vi "CRYInsert All to Listbox.vi"(11 "sAction":string) -> ()   [LabVIEW 2013]
uses:
  Global/CRYCurve Library Global.vi
panel:
  # "Insert All(Curve, Value, Result, Waveform) to Listbox"
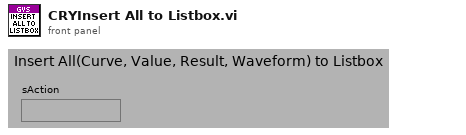
[diagram p1: front panel]
types:
  T1 = cluster{"Left Cell String":string, "Child Text":string[], "Child Tag":string, "Item Indent":i32, "Child Only?":bool, "Glyph Index":i32}[]
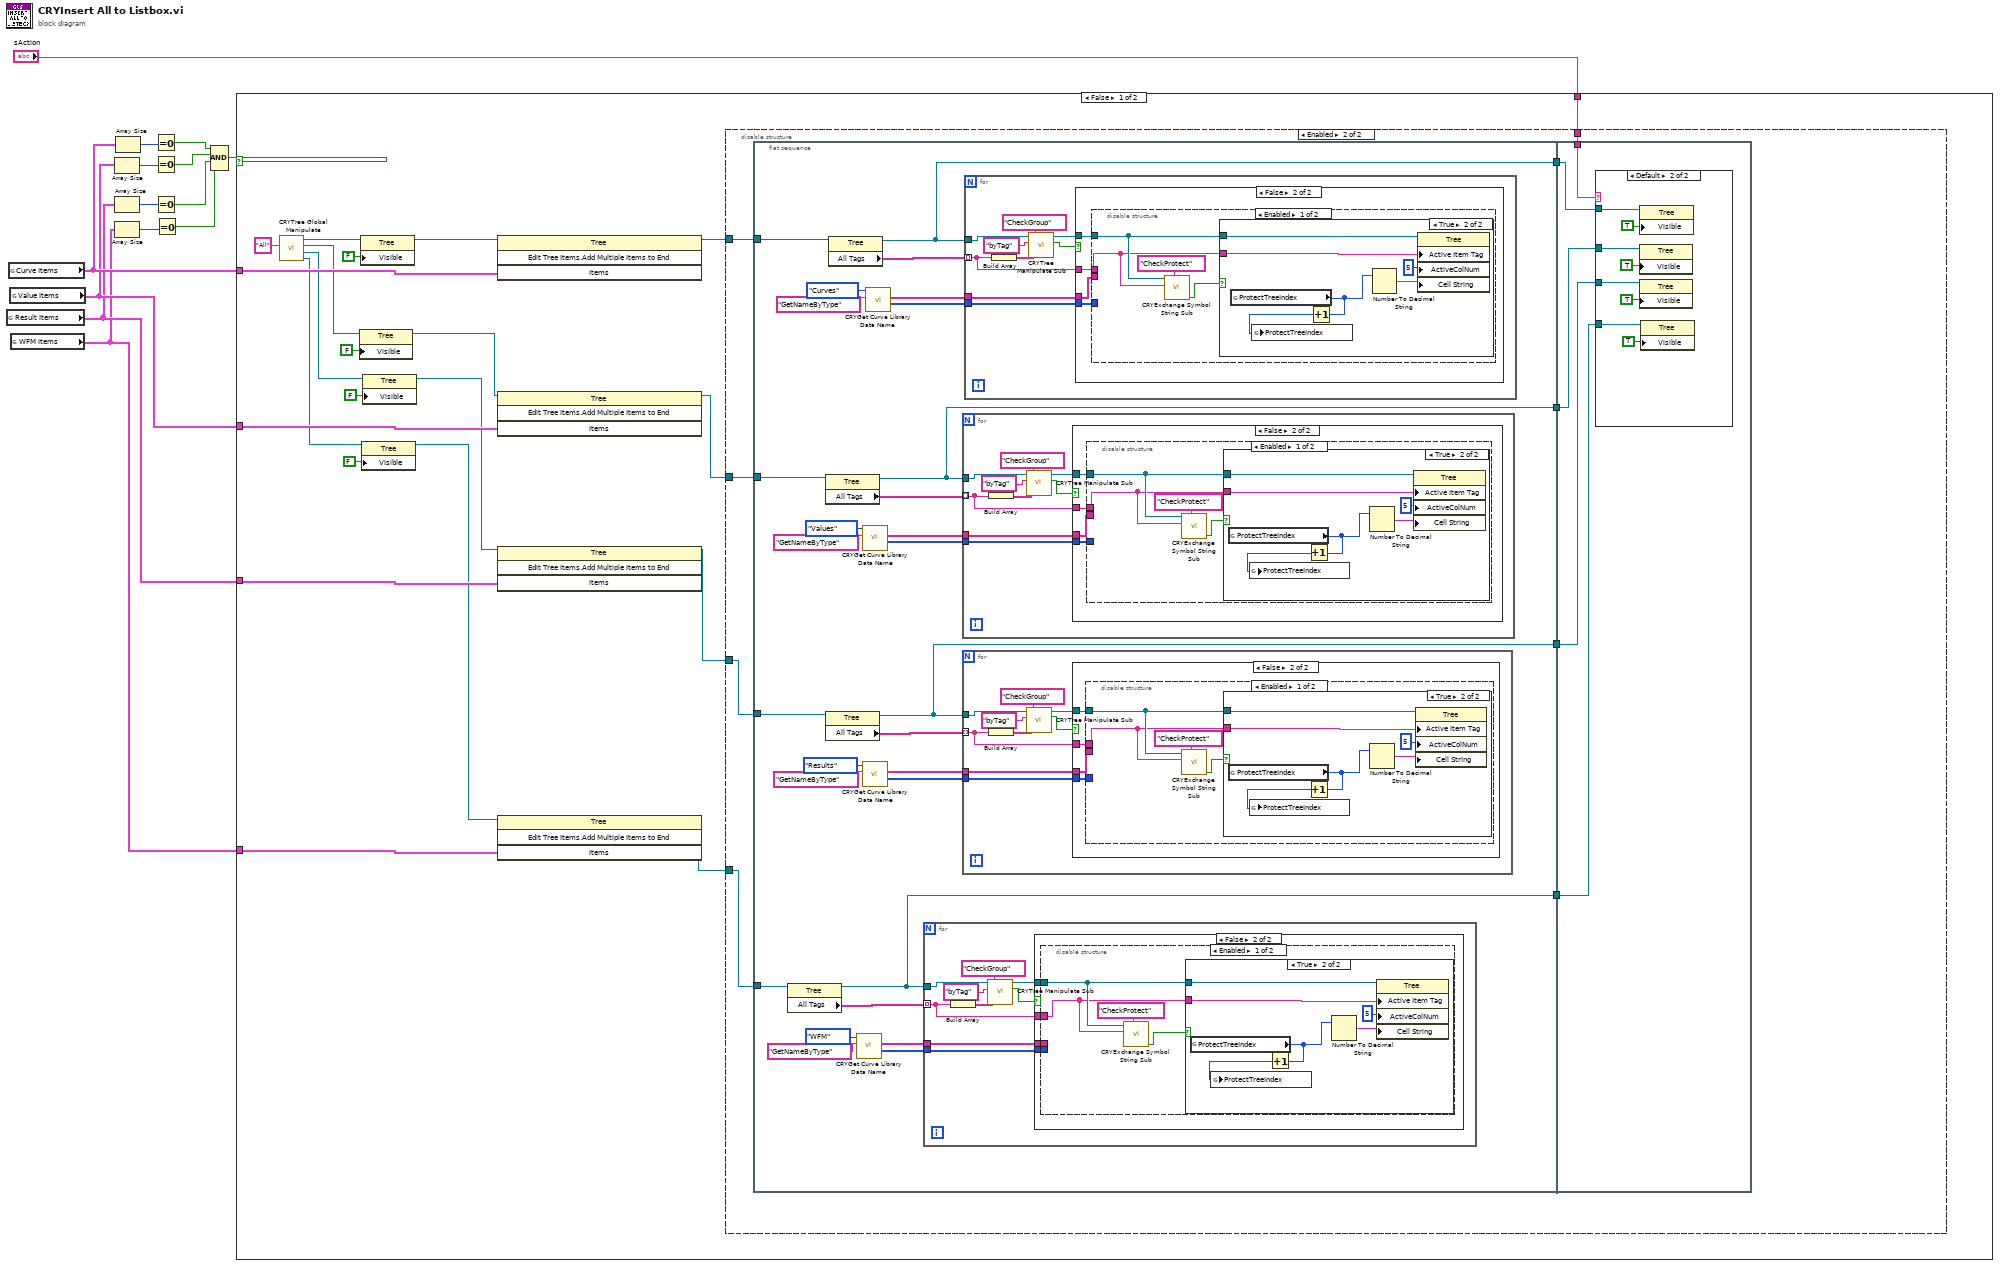
[diagram p0: block diagram]
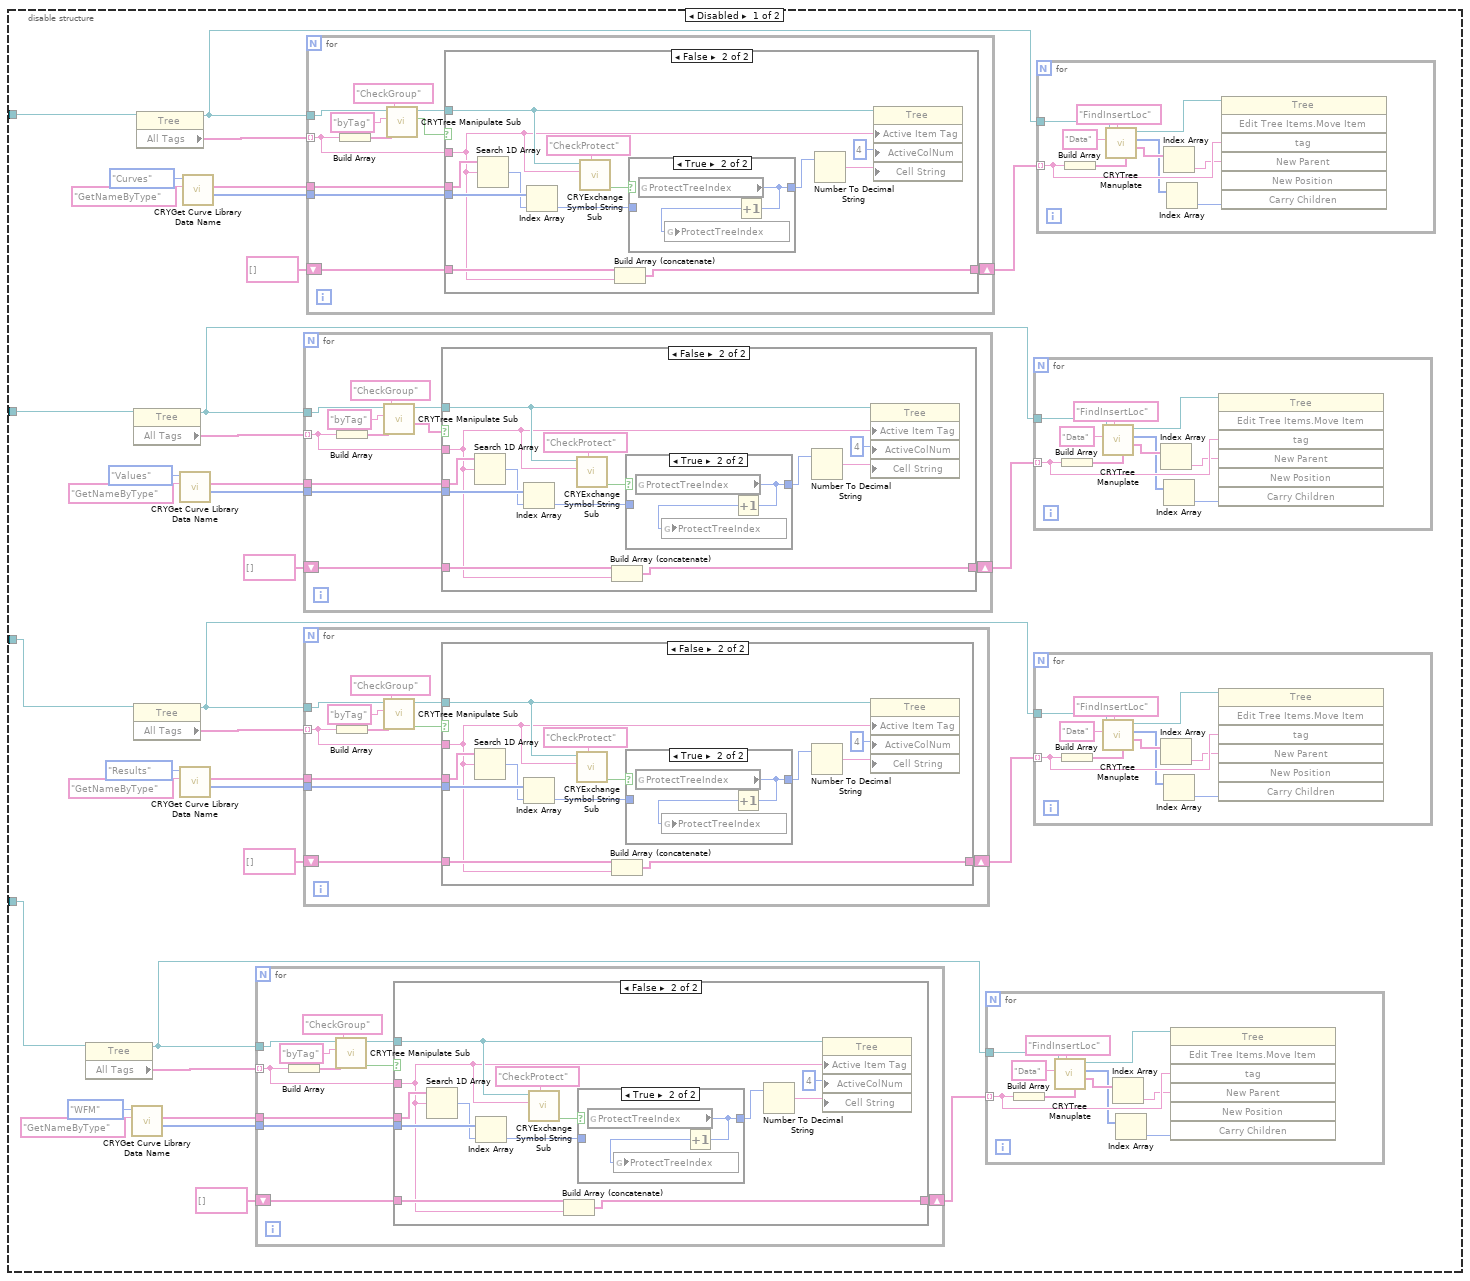
[diagram p2: hidden frame]
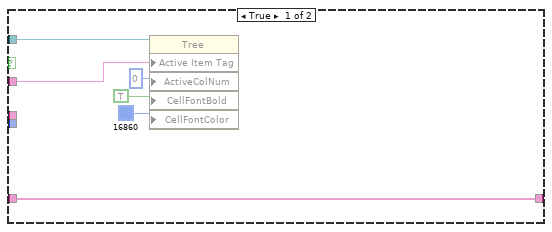
[diagram p3: hidden frame]
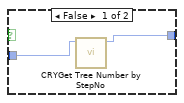
[diagram p4: hidden frame]
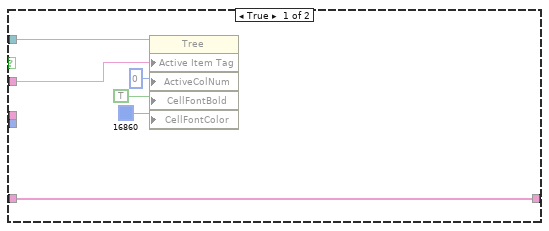
[diagram p5: hidden frame]
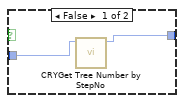
[diagram p6: hidden frame]
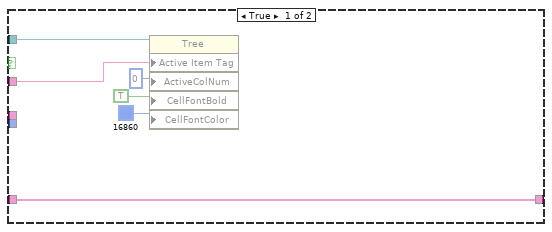
[diagram p7: hidden frame]
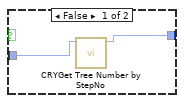
[diagram p8: hidden frame]
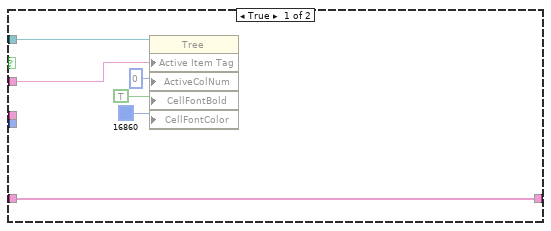
[diagram p9: hidden frame]
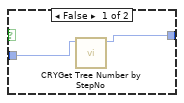
[diagram p10: hidden frame]
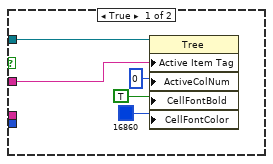
[diagram p11: hidden frame]
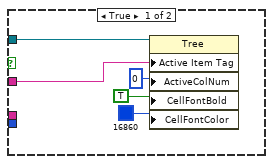
[diagram p14: hidden frame]
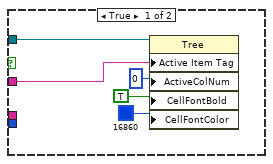
[diagram p17: hidden frame]
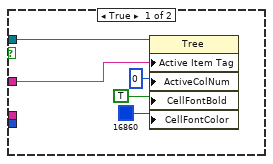
[diagram p20: hidden frame]
diagram:
  n1 = global read "CRYCurve Library Global.vi" "Result Items"() -> (w12:T1)
  n2 = global read "CRYCurve Library Global.vi" "Curve Items"() -> (w14:T1)
  n3 = global read "CRYCurve Library Global.vi" "Value Items"() -> (w13:T1)
  n4 = global read "CRYCurve Library Global.vi" "WFM Items"() -> (w11:T1)
  n5 = Array Size(array=w13) -> (size(s)=w9:i32)
  n6 = Array Size(array=w12) -> (size(s)=w8:i32)
  n7 = Array Size(array=w11) -> (size(s)=w7:i32)
  n8 = Array Size(array=w14) -> (size(s)=w10:i32)
  n9 = Equal To 0?(x=w10) -> (x = 0?=w6:bool)
  n10 = Equal To 0?(x=w9) -> (x = 0?=w4:bool)
  n11 = Equal To 0?(x=w8) -> (x = 0?=w5:bool)
  n12 = Equal To 0?(x=w7) -> (x = 0?=w3:bool)
  n13 = Compound Arithmetic op=AND(w6, w4, w5, w3) -> (w2:bool)
  n14 = case shown="False" w2 {
    tunnel: w14 -> [w31 _]
    tunnel: w13 -> [w30 _]
    tunnel: w12 -> [w29 _]
    tunnel: w11 -> [w28 _]
    tunnel: "sAction" -> [w15 _]
    frame False {
      n15 = call "CRYTree Global Manipulate.vi"("sOption"="All") -> ("WFM Tree"=w18:refnum<vi>, "Results Tree"=w20:refnum<vi>, "Values Tree"=w23:refnum<vi>, "Tree/Curve Tree"=w27:refnum<vi>)  [unwired: 7 in]
      n16 = property class="Tree"(reference=w23, "Visible"=FALSE) -> (reference out=w22:refnum<vi>)  [unwired: 1 in, 1 out]
      n17 = property class="Tree"(reference=w27, "Visible"=FALSE) -> (reference out=w26:refnum<vi>)  [unwired: 1 in, 1 out]
      n18 = property class="Tree"(reference=w18, "Visible"=FALSE) -> (reference out=w16:refnum<vi>)  [unwired: 1 in, 1 out]
      n19 = property class="Tree"(reference=w20, "Visible"=FALSE) -> (reference out=w17:refnum<vi>)  [unwired: 1 in, 1 out]
      n20 = invoke class="Tree" method="Edit Tree Items.Add Multiple Items to End"(reference=w26, "Items"=w31) -> (reference out=w36:refnum<vi>)  [unwired: 2 in, 3 out]
      n21 = invoke class="Tree" method="Edit Tree Items.Add Multiple Items to End"(reference=w22, "Items"=w30) -> (reference out=w33:refnum<vi>)  [unwired: 2 in, 3 out]
      n22 = invoke class="Tree" method="Edit Tree Items.Add Multiple Items to End"(reference=w17, "Items"=w29) -> (reference out=w34:refnum<vi>)  [unwired: 2 in, 3 out]
      n23 = invoke class="Tree" method="Edit Tree Items.Add Multiple Items to End"(reference=w16, "Items"=w28) -> (reference out=w35:refnum<vi>)  [unwired: 2 in, 3 out]
      n24 = disable-structure shown="Enabled" {
        disable-tunnel: w36 -> [w70 w257]
        disable-tunnel: w35 -> [w37 w254]
        disable-tunnel: w34 -> [w46 w255]
        disable-tunnel: w33 -> [w55 w256]
        disable-tunnel: w15 -> [_ w252]
        frame Disabled {
          n25 = property class="Tree"(reference=w37) -> (reference out=w39:refnum<vi>, "All Tags"=w40:string[])  [unwired: 1 in, 1 out]
          n26 = call "CRYGet Curve Library Data Name.vi"("sAction"="GetNameByType", "Type"=enum16{"Curves", "Values", "Results", "WFM"}."WFM") -> ("nStep No"=w43:i32[], "sNames"=w42:string[])  [unwired: 6 in, 2 out]
          n27 = property class="Tree"(reference=w55) -> (reference out=w57:refnum<vi>, "All Tags"=w58:string[])  [unwired: 1 in, 1 out]
          n28 = property class="Tree"(reference=w46) -> (reference out=w48:refnum<vi>, "All Tags"=w49:string[])  [unwired: 1 in, 1 out]
          n29 = property class="Tree"(reference=w70) -> (reference out=w71:refnum<vi>, "All Tags"=w69:string[])  [unwired: 1 in, 1 out]
          n30 = call "CRYGet Curve Library Data Name.vi"("sAction"="GetNameByType", "Type"=enum16{"Curves", "Values", "Results", "WFM"}."Values") -> ("nStep No"=w61:i32[], "sNames"=w60:string[])  [unwired: 6 in, 2 out]
          n31 = call "CRYGet Curve Library Data Name.vi"("sAction"="GetNameByType", "Type"=enum16{"Curves", "Values", "Results", "WFM"}."Results") -> ("nStep No"=w52:i32[], "sNames"=w51:string[])  [unwired: 6 in, 2 out]
          n32 = call "CRYGet Curve Library Data Name.vi"("sAction"="GetNameByType", "Type"=enum16{"Curves", "Values", "Results", "WFM"}."Curves") -> ("nStep No"=w66:i32[], "sNames"=w67:string[])  [unwired: 6 in, 2 out]
          n33 = for {
            tunnel: w40 -> [w87] mode=indexing
            tunnel: w39 -> [w91]
            tunnel: w42 -> [w86]
            tunnel: w43 -> [w85]
            shift-right: [w83] -> w38
            shift-left: string[] [] ("sNames") -> [w84]
            n34 = Build Array(w87) -> (w90:string[])
            n35 = call "CRYTree Manipulate Sub.vi"("sAction"="CheckGroup", "sData"=w90, "sOption"="byTag", "Tree in"=w91) -> ("bData out"=w89:bool, "Tree Out"=w88:refnum<vi>)  [unwired: 3 in, 3 out]
            n36 = case shown="False" w89 {
              tunnel: w88 -> [w96 w101]
              tunnel: w87 -> [w95 w100]
              tunnel: w86 -> [_ w110]
              tunnel: w85 -> [_ w109]
              tunnel: w84 -> [w94 w107]
              tunnel: [w94 w106] -> w83
              frame True {
                n37 = property class="Tree"(reference=w96, "Active Item Tag"=w95, "ActiveColNum"=0 ("Active Cell:Active Column Number"), "CellFontBold"=TRUE ("Active Cell:Cell Font:Bold"), "CellFontColor"=u32 16860) -> ()  [unwired: 1 in, 2 out]
              }
              frame False {
                n38 = Search 1D Array(1D array=w110, element=w100) -> (index of element=w108:i32)  [unwired: 1 in]
                n39 = Index Array(array=w109, index=w108) -> (element=w102:i32)
                n40 = call "CRYExchange Symbol String Sub.vi"("sAction"="CheckProtect", "sData"=w100, "Tree in"=w101) -> ("bData Out"=w105:bool)  [unwired: 5 in, 3 out]
                n41 = Build Array (concatenate)(w107, w100) -> (w106:string[])
                n42 = case shown="True" w105 {
                  tunnel: [w114 w115] -> w103
                  tunnel: w102 -> [w113 _]
                  frame False {
                    n43 = call "CRYGet Tree Number by StepNo.vi"("Step Setup VI No"=w113) -> ("Number in Tree"=w114:i32)  [unwired: 9 in, 1 out]
                  }
                  frame True {
                    n44 = global read "CRYCurve Library Global.vi" "ProtectTreeIndex"() -> (w115:i32)
                    n45 = Increment(x=w115) -> (x+1=w116:i32)
                    n46 = global write "CRYCurve Library Global.vi" "ProtectTreeIndex"(w116) -> ()
                  }
                }
                n47 = Number To Decimal String(number=w103) -> (decimal integer string=w111:string)  [unwired: 1 in]
                n48 = property class="Tree"(reference=w101, "Active Item Tag"=w100, "ActiveColNum"=4 ("Active Cell:Active Column Number"), "Cell String"=w111) -> ()  [unwired: 1 in, 2 out]
              }
            }
          }
          n49 = for {
            tunnel: w58 -> [w176] mode=indexing
            tunnel: w57 -> [w179]
            tunnel: w60 -> [w175]
            tunnel: w61 -> [w174]
            shift-right: [w172] -> w56
            shift-left: string[] [] ("sNames") -> [w173]
            n50 = Build Array(w176) -> (w178:string[])
            n51 = call "CRYTree Manipulate Sub.vi"("sAction"="CheckGroup", "sData"=w178, "sOption"="byTag", "Tree in"=w179) -> ("sData Out"=w171:string[], "Tree Out"=w177:refnum<vi>)  [unwired: 3 in, 3 out]
            n52 = case shown="False" w171 {
              tunnel: w177 -> [w184 w189]
              tunnel: w176 -> [w183 w188]
              tunnel: w175 -> [_ w198]
              tunnel: w174 -> [_ w197]
              tunnel: w173 -> [w182 w195]
              tunnel: [w182 w194] -> w172
              frame True {
                n53 = property class="Tree"(reference=w184, "Active Item Tag"=w183, "ActiveColNum"=0 ("Active Cell:Active Column Number"), "CellFontBold"=TRUE ("Active Cell:Cell Font:Bold"), "CellFontColor"=u32 16860) -> ()  [unwired: 1 in, 2 out]
              }
              frame False {
                n54 = Search 1D Array(1D array=w198, element=w188) -> (index of element=w196:i32)  [unwired: 1 in]
                n55 = Index Array(array=w197, index=w196) -> (element=w190:i32)
                n56 = call "CRYExchange Symbol String Sub.vi"("sAction"="CheckProtect", "sData"=w188, "Tree in"=w189) -> ("bData Out"=w193:bool)  [unwired: 5 in, 3 out]
                n57 = Build Array (concatenate)(w195, w188) -> (w194:string[])
                n58 = case shown="True" w193 {
                  tunnel: [w202 w203] -> w191
                  tunnel: w190 -> [w201 _]
                  frame False {
                    n59 = call "CRYGet Tree Number by StepNo.vi"("Step Setup VI No"=w201) -> ("Number in Tree"=w202:i32)  [unwired: 9 in, 1 out]
                  }
                  frame True {
                    n60 = global read "CRYCurve Library Global.vi" "ProtectTreeIndex"() -> (w203:i32)
                    n61 = Increment(x=w203) -> (x+1=w204:i32)
                    n62 = global write "CRYCurve Library Global.vi" "ProtectTreeIndex"(w204) -> ()
                  }
                }
                n63 = Number To Decimal String(number=w191) -> (decimal integer string=w199:string)  [unwired: 1 in]
                n64 = property class="Tree"(reference=w189, "Active Item Tag"=w188, "ActiveColNum"=4 ("Active Cell:Active Column Number"), "Cell String"=w199) -> ()  [unwired: 1 in, 2 out]
              }
            }
          }
          n65 = for {
            tunnel: w49 -> [w131] mode=indexing
            tunnel: w48 -> [w135]
            tunnel: w51 -> [w130]
            tunnel: w52 -> [w129]
            shift-right: [w127] -> w47
            shift-left: string[] [] ("sNames") -> [w128]
            n66 = Build Array(w131) -> (w134:string[])
            n67 = call "CRYTree Manipulate Sub.vi"("sAction"="CheckGroup", "sData"=w134, "sOption"="byTag", "Tree in"=w135) -> ("bData out"=w133:bool, "Tree Out"=w132:refnum<vi>)  [unwired: 3 in, 3 out]
            n68 = case shown="False" w133 {
              tunnel: w132 -> [w140 w145]
              tunnel: w131 -> [w139 w144]
              tunnel: w130 -> [_ w154]
              tunnel: w129 -> [_ w153]
              tunnel: w128 -> [w138 w151]
              tunnel: [w138 w150] -> w127
              frame True {
                n69 = property class="Tree"(reference=w140, "Active Item Tag"=w139, "ActiveColNum"=0 ("Active Cell:Active Column Number"), "CellFontBold"=TRUE ("Active Cell:Cell Font:Bold"), "CellFontColor"=u32 16860) -> ()  [unwired: 1 in, 2 out]
              }
              frame False {
                n70 = Search 1D Array(1D array=w154, element=w144) -> (index of element=w152:i32)  [unwired: 1 in]
                n71 = Index Array(array=w153, index=w152) -> (element=w146:i32)
                n72 = call "CRYExchange Symbol String Sub.vi"("sAction"="CheckProtect", "sData"=w144, "Tree in"=w145) -> ("bData Out"=w149:bool)  [unwired: 5 in, 3 out]
                n73 = Build Array (concatenate)(w151, w144) -> (w150:string[])
                n74 = case shown="True" w149 {
                  tunnel: [w158 w159] -> w147
                  tunnel: w146 -> [w157 _]
                  frame False {
                    n75 = call "CRYGet Tree Number by StepNo.vi"("Step Setup VI No"=w157) -> ("Number in Tree"=w158:i32)  [unwired: 9 in, 1 out]
                  }
                  frame True {
                    n76 = global read "CRYCurve Library Global.vi" "ProtectTreeIndex"() -> (w159:i32)
                    n77 = Increment(x=w159) -> (x+1=w160:i32)
                    n78 = global write "CRYCurve Library Global.vi" "ProtectTreeIndex"(w160) -> ()
                  }
                }
                n79 = Number To Decimal String(number=w147) -> (decimal integer string=w155:string)  [unwired: 1 in]
                n80 = property class="Tree"(reference=w145, "Active Item Tag"=w144, "ActiveColNum"=4 ("Active Cell:Active Column Number"), "Cell String"=w155) -> ()  [unwired: 1 in, 2 out]
              }
            }
          }
          n81 = for {
            tunnel: w69 -> [w220] mode=indexing
            tunnel: w71 -> [w223]
            tunnel: w67 -> [w219]
            tunnel: w66 -> [w218]
            shift-right: [w216] -> w72
            shift-left: string[] [] ("sNames") -> [w217]
            n82 = Build Array(w220) -> (w222:string[])
            n83 = call "CRYTree Manipulate Sub.vi"("sAction"="CheckGroup", "sData"=w222, "sOption"="byTag", "Tree in"=w223) -> ("bOnlyGroup"=w215:bool, "Tree Out"=w221:refnum<vi>)  [unwired: 3 in, 3 out]
            n84 = case shown="False" w215 {
              tunnel: w221 -> [w228 w233]
              tunnel: w220 -> [w227 w232]
              tunnel: w219 -> [_ w242]
              tunnel: w218 -> [_ w241]
              tunnel: w217 -> [w226 w239]
              tunnel: [w226 w238] -> w216
              frame True {
                n85 = property class="Tree"(reference=w228, "Active Item Tag"=w227, "ActiveColNum"=0 ("Active Cell:Active Column Number"), "CellFontBold"=TRUE ("Active Cell:Cell Font:Bold"), "CellFontColor"=u32 16860) -> ()  [unwired: 1 in, 2 out]
              }
              frame False {
                n86 = Search 1D Array(1D array=w242, element=w232) -> (index of element=w240:i32)  [unwired: 1 in]
                n87 = Index Array(array=w241, index=w240) -> (element=w234:i32)
                n88 = call "CRYExchange Symbol String Sub.vi"("sAction"="CheckProtect", "sData"=w232, "Tree in"=w233) -> ("bData Out"=w237:bool)  [unwired: 5 in, 3 out]
                n89 = Build Array (concatenate)(w239, w232) -> (w238:string[])
                n90 = case shown="True" w237 {
                  tunnel: [w246 w247] -> w235
                  tunnel: w234 -> [w245 _]
                  frame False {
                    n91 = call "CRYGet Tree Number by StepNo.vi"("Step Setup VI No"=w245) -> ("Number in Tree"=w246:i32)  [unwired: 9 in, 1 out]
                  }
                  frame True {
                    n92 = global read "CRYCurve Library Global.vi" "ProtectTreeIndex"() -> (w247:i32)
                    n93 = Increment(x=w247) -> (x+1=w248:i32)
                    n94 = global write "CRYCurve Library Global.vi" "ProtectTreeIndex"(w248) -> ()
                  }
                }
                n95 = Number To Decimal String(number=w235) -> (decimal integer string=w243:string)  [unwired: 1 in]
                n96 = property class="Tree"(reference=w233, "Active Item Tag"=w232, "ActiveColNum"=4 ("Active Cell:Active Column Number"), "Cell String"=w243) -> ()  [unwired: 1 in, 2 out]
              }
            }
          }
          n97 = for {
            tunnel: w38 -> [w77] mode=indexing
            tunnel: w39 -> [w79]
            n98 = Build Array(w77) -> (w80:string[])
            n99 = call "CRYTree Manuplate.vi"("sData"=w80, "sAction"="FindInsertLoc", "sOption"="Data", "Tree in"=w79) -> ("sData Out"=w76:string[], "nData Out"=w74:i32[], "Tree Out"=w78:refnum<vi>)  [unwired: 4 in, 1 out]
            n100 = Index Array(array=w76) -> (element=w75:string)  [unwired: 1 in]
            n101 = Index Array(array=w74) -> (element=w73:i32)  [unwired: 1 in]
            n102 = invoke class="Tree" method="Edit Tree Items.Move Item"(reference=w78, "tag"=w77, "New Parent"=w75, "New Position"=w73) -> ()  [unwired: 3 in, 7 out]
          }
          n103 = for {
            tunnel: w56 -> [w165] mode=indexing
            tunnel: w57 -> [w167]
            n104 = Build Array(w165) -> (w168:string[])
            n105 = call "CRYTree Manuplate.vi"("sData"=w168, "sAction"="FindInsertLoc", "sOption"="Data", "Tree in"=w167) -> ("sData Out"=w164:string[], "nData Out"=w162:i32[], "Tree Out"=w166:refnum<vi>)  [unwired: 4 in, 1 out]
            n106 = Index Array(array=w164) -> (element=w163:string)  [unwired: 1 in]
            n107 = Index Array(array=w162) -> (element=w161:i32)  [unwired: 1 in]
            n108 = invoke class="Tree" method="Edit Tree Items.Move Item"(reference=w166, "tag"=w165, "New Parent"=w163, "New Position"=w161) -> ()  [unwired: 3 in, 7 out]
          }
          n109 = for {
            tunnel: w47 -> [w121] mode=indexing
            tunnel: w48 -> [w123]
            n110 = Build Array(w121) -> (w124:string[])
            n111 = call "CRYTree Manuplate.vi"("sData"=w124, "sAction"="FindInsertLoc", "sOption"="Data", "Tree in"=w123) -> ("sData Out"=w120:string[], "nData Out"=w118:i32[], "Tree Out"=w122:refnum<vi>)  [unwired: 4 in, 1 out]
            n112 = Index Array(array=w120) -> (element=w119:string)  [unwired: 1 in]
            n113 = Index Array(array=w118) -> (element=w117:i32)  [unwired: 1 in]
            n114 = invoke class="Tree" method="Edit Tree Items.Move Item"(reference=w122, "tag"=w121, "New Parent"=w119, "New Position"=w117) -> ()  [unwired: 3 in, 7 out]
          }
          n115 = for {
            tunnel: w72 -> [w209] mode=indexing
            tunnel: w71 -> [w211]
            n116 = Build Array(w209) -> (w212:string[])
            n117 = call "CRYTree Manuplate.vi"("sData"=w212, "sAction"="FindInsertLoc", "sOption"="Data", "Tree in"=w211) -> ("sData Out"=w208:string[], "nData Out"=w206:i32[], "Tree Out"=w210:refnum<vi>)  [unwired: 4 in, 1 out]
            n118 = Index Array(array=w208) -> (element=w207:string)  [unwired: 1 in]
            n119 = Index Array(array=w206) -> (element=w205:i32)  [unwired: 1 in]
            n120 = invoke class="Tree" method="Edit Tree Items.Move Item"(reference=w210, "tag"=w209, "New Parent"=w207, "New Position"=w205) -> ()  [unwired: 3 in, 7 out]
          }
        }
        frame Enabled {
          n121 = flat-sequence {
            tunnel: w257 -> [w285]
            tunnel: w256 -> [w274]
            tunnel: w255 -> [w268]
            tunnel: w254 -> [w262]
            tunnel: [w261] -> w253
            tunnel: [w260] -> w251
            tunnel: [w259] -> w250
            tunnel: [w258] -> w249
            tunnel: w253 -> [w401]
            tunnel: w252 -> [w402]
            tunnel: w251 -> [w400]
            tunnel: w250 -> [w399]
            tunnel: w249 -> [w398]
            frame #0 {
              n122 = property class="Tree"(reference=w262) -> (reference out=w258:refnum<vi>, "All Tags"=w263:string[])  [unwired: 1 in, 1 out]
              n123 = property class="Tree"(reference=w274) -> (reference out=w260:refnum<vi>, "All Tags"=w275:string[])  [unwired: 1 in, 1 out]
              n124 = property class="Tree"(reference=w268) -> (reference out=w259:refnum<vi>, "All Tags"=w269:string[])  [unwired: 1 in, 1 out]
              n125 = property class="Tree"(reference=w285) -> (reference out=w261:refnum<vi>, "All Tags"=w284:string[])  [unwired: 1 in, 1 out]
              n126 = call "CRYGet Curve Library Data Name.vi"("sAction"="GetNameByType", "Type"=enum16{"Curves", "Values", "Results", "WFM"}."WFM") -> ("nStep No"=w266:i32[], "sNames"=w265:string[])  [unwired: 6 in, 2 out]
              n127 = call "CRYGet Curve Library Data Name.vi"("sAction"="GetNameByType", "Type"=enum16{"Curves", "Values", "Results", "WFM"}."Values") -> ("nStep No"=w278:i32[], "sNames"=w277:string[])  [unwired: 6 in, 2 out]
              n128 = call "CRYGet Curve Library Data Name.vi"("sAction"="GetNameByType", "Type"=enum16{"Curves", "Values", "Results", "WFM"}."Results") -> ("nStep No"=w272:i32[], "sNames"=w271:string[])  [unwired: 6 in, 2 out]
              n129 = call "CRYGet Curve Library Data Name.vi"("sAction"="GetNameByType", "Type"=enum16{"Curves", "Values", "Results", "WFM"}."Curves") -> ("nStep No"=w281:i32[], "sNames"=w282:string[])  [unwired: 6 in, 2 out]
              n130 = for {
                tunnel: w263 -> [w289] mode=indexing
                tunnel: w258 -> [w292]
                tunnel: w265 -> [w288]
                tunnel: w266 -> [w287]
                n131 = Build Array(w289) -> (w291:string[])
                n132 = call "CRYTree Manipulate Sub.vi"("sAction"="CheckGroup", "sData"=w291, "sOption"="byTag", "Tree in"=w292) -> ("bOnlyGroup"=w286:bool, "Tree Out"=w290:refnum<vi>)  [unwired: 3 in, 3 out]
                n133 = case shown="False" w286 {
                  tunnel: w290 -> [w296 w301]
                  tunnel: w289 -> [w295 w300]
                  tunnel: w288 -> [_ w303]
                  tunnel: w287 -> [_ w302]
                  frame True {
                    n134 = property class="Tree"(reference=w296, "Active Item Tag"=w295, "ActiveColNum"=0 ("Active Cell:Active Column Number"), "CellFontBold"=TRUE ("Active Cell:Cell Font:Bold"), "CellFontColor"=u32 16860) -> ()  [unwired: 1 in, 2 out]
                  }
                  frame False {
                    n135 = disable-structure shown="Enabled" {
                      disable-tunnel: w303 -> [_ _]
                      disable-tunnel: w302 -> [_ _]
                      disable-tunnel: w301 -> [w306 _]
                      disable-tunnel: w300 -> [w305 _]
                      frame Enabled {
                        n136 = call "CRYExchange Symbol String Sub.vi"("sAction"="CheckProtect", "sData"=w305, "Tree in"=w306) -> ("bData Out"=w304:bool)  [unwired: 5 in, 3 out]
                        n137 = case shown="True" w304 {
                          tunnel: w306 -> [_ w310]
                          tunnel: w305 -> [_ w309]
                          frame False {
                          }
                          frame True {
                            n138 = global read "CRYCurve Library Global.vi" "ProtectTreeIndex"() -> (w311:i32)
                            n139 = Increment(x=w311) -> (x+1=w308:i32)
                            n140 = global write "CRYCurve Library Global.vi" "ProtectTreeIndex"(w308) -> ()
                            n141 = Number To Decimal String(number=w311) -> (decimal integer string=w312:string)  [unwired: 1 in]
                            n142 = property class="Tree"(reference=w310, "Active Item Tag"=w309, "ActiveColNum"=5 ("Active Cell:Active Column Number"), "Cell String"=w312) -> ()  [unwired: 1 in, 2 out]
                          }
                        }
                      }
                      frame Disabled {
                      }
                    }
                  }
                }
              }
              n143 = for {
                tunnel: w275 -> [w345] mode=indexing
                tunnel: w260 -> [w348]
                tunnel: w277 -> [w344]
                tunnel: w278 -> [w343]
                n144 = Build Array(w345) -> (w347:string[])
                n145 = call "CRYTree Manipulate Sub.vi"("sAction"="CheckGroup", "sData"=w347, "sOption"="byTag", "Tree in"=w348) -> ("bOnlyGroup"=w342:bool, "Tree Out"=w346:refnum<vi>)  [unwired: 3 in, 3 out]
                n146 = case shown="False" w342 {
                  tunnel: w346 -> [w352 w357]
                  tunnel: w345 -> [w351 w356]
                  tunnel: w344 -> [_ w359]
                  tunnel: w343 -> [_ w358]
                  frame True {
                    n147 = property class="Tree"(reference=w352, "Active Item Tag"=w351, "ActiveColNum"=0 ("Active Cell:Active Column Number"), "CellFontBold"=TRUE ("Active Cell:Cell Font:Bold"), "CellFontColor"=u32 16860) -> ()  [unwired: 1 in, 2 out]
                  }
                  frame False {
                    n148 = disable-structure shown="Enabled" {
                      disable-tunnel: w359 -> [_ _]
                      disable-tunnel: w358 -> [_ _]
                      disable-tunnel: w357 -> [w362 _]
                      disable-tunnel: w356 -> [w361 _]
                      frame Enabled {
                        n149 = call "CRYExchange Symbol String Sub.vi"("sAction"="CheckProtect", "sData"=w361, "Tree in"=w362) -> ("bData Out"=w360:bool)  [unwired: 5 in, 3 out]
                        n150 = case shown="True" w360 {
                          tunnel: w362 -> [_ w366]
                          tunnel: w361 -> [_ w365]
                          frame False {
                          }
                          frame True {
                            n151 = global read "CRYCurve Library Global.vi" "ProtectTreeIndex"() -> (w367:i32)
                            n152 = Increment(x=w367) -> (x+1=w364:i32)
                            n153 = global write "CRYCurve Library Global.vi" "ProtectTreeIndex"(w364) -> ()
                            n154 = Number To Decimal String(number=w367) -> (decimal integer string=w368:string)  [unwired: 1 in]
                            n155 = property class="Tree"(reference=w366, "Active Item Tag"=w365, "ActiveColNum"=5 ("Active Cell:Active Column Number"), "Cell String"=w368) -> ()  [unwired: 1 in, 2 out]
                          }
                        }
                      }
                      frame Disabled {
                      }
                    }
                  }
                }
              }
              n156 = for {
                tunnel: w269 -> [w317] mode=indexing
                tunnel: w259 -> [w320]
                tunnel: w271 -> [w316]
                tunnel: w272 -> [w315]
                n157 = Build Array(w317) -> (w319:string[])
                n158 = call "CRYTree Manipulate Sub.vi"("sAction"="CheckGroup", "sData"=w319, "sOption"="byTag", "Tree in"=w320) -> ("bOnlyGroup"=w314:bool, "Tree Out"=w318:refnum<vi>)  [unwired: 3 in, 3 out]
                n159 = case shown="False" w314 {
                  tunnel: w318 -> [w324 w329]
                  tunnel: w317 -> [w323 w328]
                  tunnel: w316 -> [_ w331]
                  tunnel: w315 -> [_ w330]
                  frame True {
                    n160 = property class="Tree"(reference=w324, "Active Item Tag"=w323, "ActiveColNum"=0 ("Active Cell:Active Column Number"), "CellFontBold"=TRUE ("Active Cell:Cell Font:Bold"), "CellFontColor"=u32 16860) -> ()  [unwired: 1 in, 2 out]
                  }
                  frame False {
                    n161 = disable-structure shown="Enabled" {
                      disable-tunnel: w331 -> [_ _]
                      disable-tunnel: w330 -> [_ _]
                      disable-tunnel: w329 -> [w334 _]
                      disable-tunnel: w328 -> [w333 _]
                      frame Enabled {
                        n162 = call "CRYExchange Symbol String Sub.vi"("sAction"="CheckProtect", "sData"=w333, "Tree in"=w334) -> ("bData Out"=w332:bool)  [unwired: 5 in, 3 out]
                        n163 = case shown="True" w332 {
                          tunnel: w334 -> [_ w338]
                          tunnel: w333 -> [_ w337]
                          frame False {
                          }
                          frame True {
                            n164 = global read "CRYCurve Library Global.vi" "ProtectTreeIndex"() -> (w339:i32)
                            n165 = Increment(x=w339) -> (x+1=w336:i32)
                            n166 = global write "CRYCurve Library Global.vi" "ProtectTreeIndex"(w336) -> ()
                            n167 = Number To Decimal String(number=w339) -> (decimal integer string=w340:string)  [unwired: 1 in]
                            n168 = property class="Tree"(reference=w338, "Active Item Tag"=w337, "ActiveColNum"=5 ("Active Cell:Active Column Number"), "Cell String"=w340) -> ()  [unwired: 1 in, 2 out]
                          }
                        }
                      }
                      frame Disabled {
                      }
                    }
                  }
                }
              }
              n169 = for {
                tunnel: w284 -> [w373] mode=indexing
                tunnel: w261 -> [w376]
                tunnel: w282 -> [w372]
                tunnel: w281 -> [w371]
                n170 = Build Array(w373) -> (w375:string[])
                n171 = call "CRYTree Manipulate Sub.vi"("sAction"="CheckGroup", "sData"=w375, "sOption"="byTag", "Tree in"=w376) -> ("bOnlyGroup"=w370:bool, "Tree Out"=w374:refnum<vi>)  [unwired: 3 in, 3 out]
                n172 = case shown="False" w370 {
                  tunnel: w374 -> [w380 w385]
                  tunnel: w373 -> [w379 w384]
                  tunnel: w372 -> [_ w387]
                  tunnel: w371 -> [_ w386]
                  frame True {
                    n173 = property class="Tree"(reference=w380, "Active Item Tag"=w379, "ActiveColNum"=0 ("Active Cell:Active Column Number"), "CellFontBold"=TRUE ("Active Cell:Cell Font:Bold"), "CellFontColor"=u32 16860) -> ()  [unwired: 1 in, 2 out]
                  }
                  frame False {
                    n174 = disable-structure shown="Enabled" {
                      disable-tunnel: w387 -> [_ _]
                      disable-tunnel: w386 -> [_ _]
                      disable-tunnel: w385 -> [w390 _]
                      disable-tunnel: w384 -> [w389 _]
                      frame Enabled {
                        n175 = call "CRYExchange Symbol String Sub.vi"("sAction"="CheckProtect", "sData"=w389, "Tree in"=w390) -> ("bData Out"=w388:bool)  [unwired: 5 in, 3 out]
                        n176 = case shown="True" w388 {
                          tunnel: w390 -> [_ w394]
                          tunnel: w389 -> [_ w393]
                          frame False {
                          }
                          frame True {
                            n177 = global read "CRYCurve Library Global.vi" "ProtectTreeIndex"() -> (w395:i32)
                            n178 = Increment(x=w395) -> (x+1=w392:i32)
                            n179 = global write "CRYCurve Library Global.vi" "ProtectTreeIndex"(w392) -> ()
                            n180 = Number To Decimal String(number=w395) -> (decimal integer string=w396:string)  [unwired: 1 in]
                            n181 = property class="Tree"(reference=w394, "Active Item Tag"=w393, "ActiveColNum"=5 ("Active Cell:Active Column Number"), "Cell String"=w396) -> ()  [unwired: 1 in, 2 out]
                          }
                        }
                      }
                      frame Disabled {
                      }
                    }
                  }
                }
              }
            }
            frame #1 {
              n182 = case shown="Default" w402 {
                tunnel: w401 -> [_ w409]
                tunnel: w400 -> [_ w405]
                tunnel: w399 -> [_ w404]
                tunnel: w398 -> [_ w403]
                frame "Invisible" {
                }
                frame Default {
                  n183 = property class="Tree"(reference=w405, "Visible"=TRUE) -> ()  [unwired: 1 in, 2 out]
                  n184 = property class="Tree"(reference=w404, "Visible"=TRUE) -> ()  [unwired: 1 in, 2 out]
                  n185 = property class="Tree"(reference=w409, "Visible"=TRUE) -> ()  [unwired: 1 in, 2 out]
                  n186 = property class="Tree"(reference=w403, "Visible"=TRUE) -> ()  [unwired: 1 in, 2 out]
                }
              }
            }
          }
        }
      }
    }
    frame True {
      n187 = call "CRYInsert All to Listbox Etc.vi"("sAction"="NewProject") -> ()  [unwired: 11 in]
    }
  }
